vi "Create New Test Case.vi"(8 "error in (no error)":errorcluster, 10 "Path":path, 11 "Application":refnum<vi>) -> (0 "error out":errorcluster)   [LabVIEW 2020, in "Project Provider.lvlib"]
uses:
  Project Provider.lvlib
  <vilib>/Utility/sysdir.llb/System Directory Type.ctl
  <vilib>/Utility/error.llb/Error Cluster From Error Code.vi
  <vilib>/ErrorRing/Error Ring.xnode
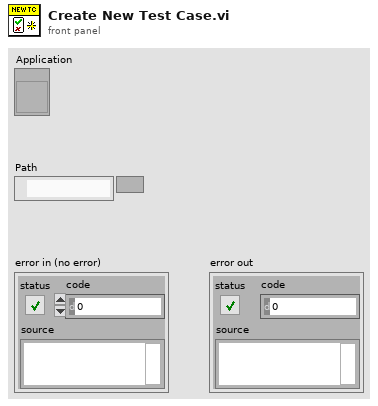
[diagram p1: front panel]
types:
  T1 = typedef "System Directory Type.ctl" = i32
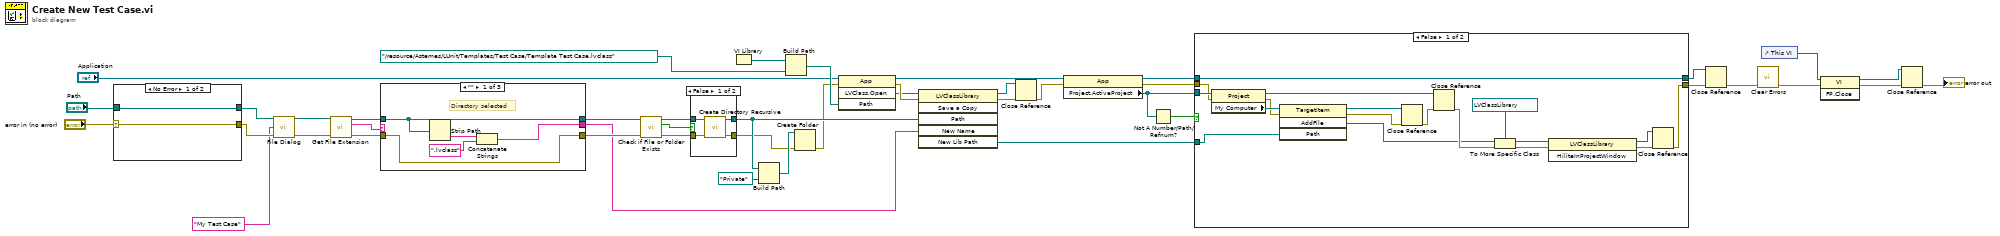
[diagram p0: block diagram]
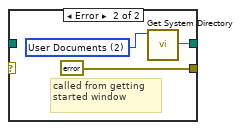
[diagram p2: hidden frame]
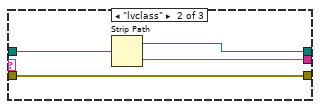
[diagram p3: hidden frame]
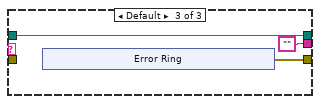
[diagram p4: hidden frame]
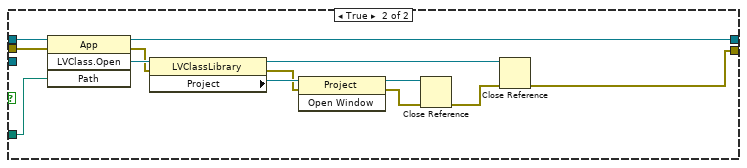
[diagram p6: hidden frame]
diagram:
  n1 = case shown="No Error" "error in (no error)" {
    selector: "error in (no error)" -> [w46 _]
    tunnel: [w46 errorcluster {"status"=FALSE, "code"=0, "source"=""} ("error IO")] -> w10
    tunnel: [w45 w47] -> w11
    tunnel: "Path" -> [w45 _]
    frame No Error {
    }
    frame Error {
      w48 = T1 2 items=["User Home"=0, "User Desktop"=1, "User Documents"=2, "User Application Data"=3, "User Preferences"=4, "User Temporary"=5, "Public Documents"=6, "Public Application Data"=7, "Public Preferences"=8, "Public Cache"=13, "System Core Libraries"=9, "System Installed Libraries"=10, "Application Files"=11, "Boot Volume Root"=12] ("system directory type")
      # "called from getting started window"
      n2 = call <vilib>:"Get System Directory.vi"("system directory type"=w48) -> ("system directory"=w47:path)  [unwired: 10 in]
    }
  }
  n3 = call "File Dialog"("start path"=w11, "default name"="My Test Case", "error in"=w10) -> ("selected path"=w41:path, "error out"=w9:errorcluster)  [unwired: 9 in, 2 out]
  n4 = call <vilib>:"Get File Extension.vi"("error in (no error)"=w9, "file"=w41) -> ("error out"=w44:errorcluster, "lowercase file extension"=w43:string, "dup file"=w42:path)  [unwired: 5 in, 2 out]
  n5 = case shown="\"\"" w43 {
    tunnel: w44 -> [w50 w55 _]
    tunnel: w42 -> [w51 w58 w59]
    tunnel: [w50 w55 w61] -> w39
    tunnel: [w52 w57 "" ("name")] -> w35
    tunnel: [w51 w56 w59] -> w40
    frame "" {
      # "Directory selected"
      n6 = Strip Path(path=w51) -> (name=w54:string)  [unwired: 1 out]
      n7 = Concatenate Strings(w54, ".lvclass" ("string")) -> (w52:string)
    }
    frame "lvclass" {
      n8 = Strip Path(path=w58) -> (stripped path=w56:path, name=w57:string)
    }
    frame Default {
      n9 = xnode "Error Ring"() -> ("error out"=w61:errorcluster)
    }
  }
  n10 = call <vilib>:"Check if File or Folder Exists.vi"("error in (no error)"=w39, "path"=w40) -> ("error out"=w38:errorcluster, "file or folder exists?"=w36:bool, "dup path"=w37:path)  [unwired: 7 in]
  n11 = case shown="False" w36 {
    tunnel: w38 -> [w69 w70]
    tunnel: w37 -> [w68 w71]
    tunnel: [w67 w71] -> w3
    tunnel: [w66 w70] -> w2
    frame False {
      n12 = call <vilib>:"Create Directory Recursive.vi"("error in (no error)"=w69, "directory"=w68) -> ("error out"=w66:errorcluster, "directory copy"=w67:path)  [unwired: 3 in, 1 out]
    }
    frame True {
    }
  }
  n13 = VI Library() -> (path=w26:path)
  n14 = Build Path(base path=w3, name or relative path=path "Private") -> (appended path=w5:path)
  n15 = Build Path(base path=w26, name or relative path=path "../resource/Astemes/LUnit/Templates/Test Case/Template Test Case.lvclass") -> (appended path=w24:path)
  n16 = Create Folder(path (use dialog)=w5, error in=w2) -> (error out=w1:errorcluster)  [unwired: 1 in, 2 out]
  n17 = invoke class="App" method="LVClass.Open"(reference="Application", error in=w1, "Path"=w24) -> (reference out=w21:refnum<vi>, error out=w34:errorcluster, "LVClass.Open"=w16:refnum<vi>)  [unwired: 1 in, 1 out]
  n18 = invoke class="LVClassLibrary" method="Save a Copy"(reference=w16, error in=w34, "Path"=w3, "New Name"=w35) -> (reference out=w22:refnum<vi>, error out=w20:errorcluster, "New Lib Path"=w30:path)  [unwired: 2 in, 3 out]
  n19 = Close Reference(reference=w22, error in (no error)=w20) -> (error out=w19:errorcluster)
  n20 = property class="App"(reference=w21, error in=w19) -> (reference out=w29:refnum<vi>, error out=w31:errorcluster, "Project.ActiveProject"=w32:refnum<vi>)
  n21 = Not A Number/Path/Refnum?(number/path/refnum=w32) -> (NaN/Path/Refnum?=w33:bool)
  n22 = case shown="False" w33 {
    tunnel: w32 -> [w89 _]
    tunnel: w31 -> [w87 w93]
    tunnel: w30 -> [w81 w91]
    tunnel: [w76 w90] -> w27
    tunnel: w29 -> [w80 w94]
    tunnel: [w80 w92] -> w28
    frame False {
      n23 = property class="Project"(reference=w89, error in=w87) -> (reference out=w83:refnum<vi>, error out=w86:errorcluster, "My Computer"=w88:refnum<vi>)
      n24 = invoke class="TargetItem" method="AddFile"(reference=w88, error in=w86, "Path"=w81) -> (reference out=w84:refnum<vi>, error out=w85:errorcluster, "AddFile"=w72:refnum<vi>)  [unwired: 1 in, 1 out]
      n25 = Close Reference(reference=w84, error in (no error)=w85) -> (error out=w82:errorcluster)
      n26 = Close Reference(reference=w83, error in (no error)=w82) -> (error out=w79:errorcluster)
      n27 = To More Specific Class(target class=refnum<vi> refnum ("reference"), reference=w72, error in=w79) -> (specific class reference=w73:refnum<vi>, error out=w75:errorcluster)
      n28 = invoke class="LVClassLibrary" method="HiliteInProjectWindow"(reference=w73, error in=w75) -> (reference out=w77:refnum<vi>, error out=w78:errorcluster)  [unwired: 1 in, 1 out]
      n29 = Close Reference(reference=w77, error in (no error)=w78) -> (error out=w76:errorcluster)
    }
    frame True {
      n30 = invoke class="App" method="LVClass.Open"(reference=w94, error in=w93, "Path"=w91) -> (reference out=w92:refnum<vi>, error out=w101:errorcluster, "LVClass.Open"=w102:refnum<vi>)  [unwired: 1 in, 1 out]
      n31 = property class="LVClassLibrary"(reference=w102, error in=w101) -> (reference out=w100:refnum<vi>, error out=w98:errorcluster, "Project"=w99:refnum<vi>)
      n32 = invoke class="Project" method="Open Window"(reference=w99, error in=w98) -> (reference out=w97:refnum<vi>, error out=w96:errorcluster)  [unwired: 1 in, 1 out]
      n33 = Close Reference(reference=w97, error in (no error)=w96) -> (error out=w95:errorcluster)
      n34 = Close Reference(reference=w100, error in (no error)=w95) -> (error out=w90:errorcluster)
    }
  }
  n35 = Close Reference(reference=w28, error in (no error)=w27) -> (error out=w23:errorcluster)
  n36 = call <vilib>:"Clear Errors.vi"("error in (no error)"=w23) -> ("error out"=w13:errorcluster)  [unwired: 5 in, 1 out]
  n37 = control-ref of="This VI"() -> (w18:refnum<vi>)
  n38 = invoke class="VI" method="FP.Close"(reference=w18, error in=w13) -> (reference out=w15:refnum<vi>, error out=w14:errorcluster)  [unwired: 1 in, 1 out]
  n39 = Close Reference(reference=w15, error in (no error)=w14) -> (error out=→"error out":errorcluster)
